vi "Read CRT.vi"(8 "error in (no error)":errorcluster, 11 "EVI 79 in":refnum<class "EVI 79.lvclass">) -> (0 "error out":errorcluster, 2 "CRT":cluster{"V":dbl, "I":dbl, "CRT_MAX_ms":dbl}={"V"=24.0, "I"=0.5, "CRT_MAX_ms"=100.0}, 3 "EVI 79 out":refnum<class "EVI 79.lvclass">)   [LabVIEW 2025, in "EVI 79.lvclass"]
uses:
  EVI 79.lvclass
  EVI 79.lvclass/EVI 79.ctl
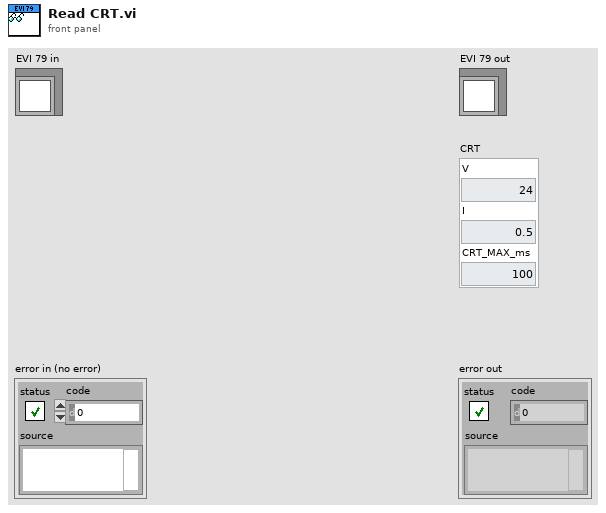
[diagram p1: front panel]
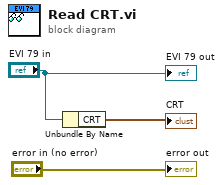
[diagram p0: block diagram]
diagram:
  n1 = Unbundle By Name("EVI 79 in") -> ("CRT"=→"CRT":cluster{"V":dbl, "I":dbl, "CRT_MAX_ms":dbl})
  "error out" <- "error in (no error)"
  "EVI 79 out" <- "EVI 79 in"
